vi "PKG_IMC_OpenX.vi"(7 "openMode":i32, 9 "timeout":i32, 10 "imcid":i32, 11 "netcardsel":i32) -> (3 "function return":u32)   [LabVIEW 2011, in "IMC_Pkg4xxx.lvlib"]
doc: "PKG_IMC_OpenX (int netcardsel, int imcid, int timeout, int openMode) ;"
uses:
  IMC_Pkg4xxx.lvlib
  IMC_Pkg4xxx.dll
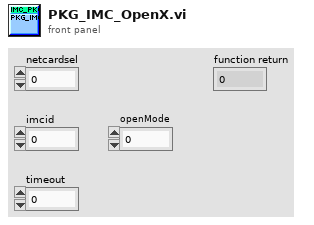
[diagram p1: front panel]
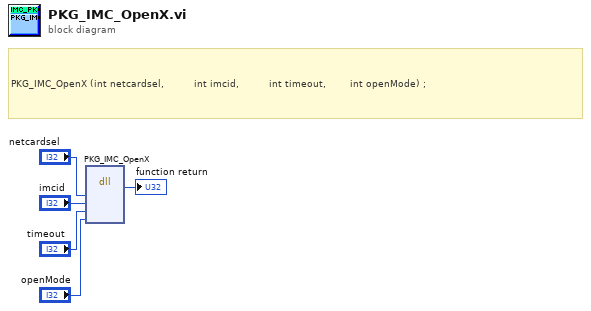
[diagram p0: block diagram]
diagram:
  # "PKG_IMC_OpenX (int netcardsel, \t\t\t\t\t\t\t\t\tint imcid, \t\t\t\t\t\t\t\t\tint timeout,\t\t\t\t\t\t\t\tint openMode) ;"
  n1 = dll-call lib="PTH1mabs F光盘刻录\niMC MotionIMCNet_V4.0IMCAppincLabviewIMC_PKG4xxxIMC_PKG4xxx\nIMC_Pkg4xxx.*" fn="PKG_IMC_OpenX"("netcardsel"="netcardsel", "imcid"="imcid", "timeout"="timeout", "openMode"="openMode") -> (→"function return":u32)  [unwired: 7 in, 2 out]
